vi "readpdf_8.6.vi"(2 "error in (no error)":errorcluster, 3 "Path":path=path "D:/dTemp/Hello World.pdf") -> (0 "error out":errorcluster, 1 "src":string)   [LabVIEW 2012]
uses:
  C:/Users/jlarrieux/Documents/Labview Git Repo/Labview Toolbox/PDFBox.NET-1.7.0/bin/pdfbox-1.7.0.dll
  PDFBox.NET-1.7.0/bin/pdfbox-1.7.0.dll
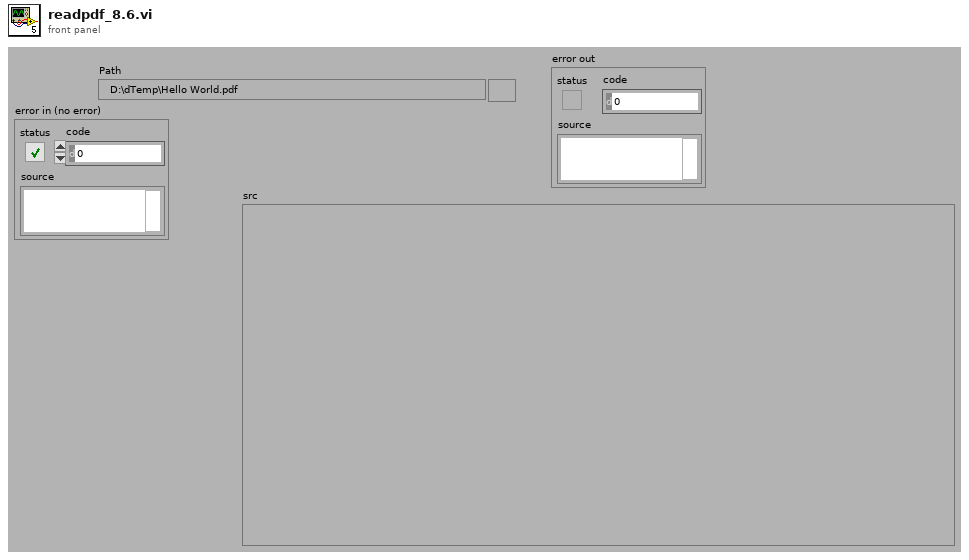
[diagram p1: front panel]
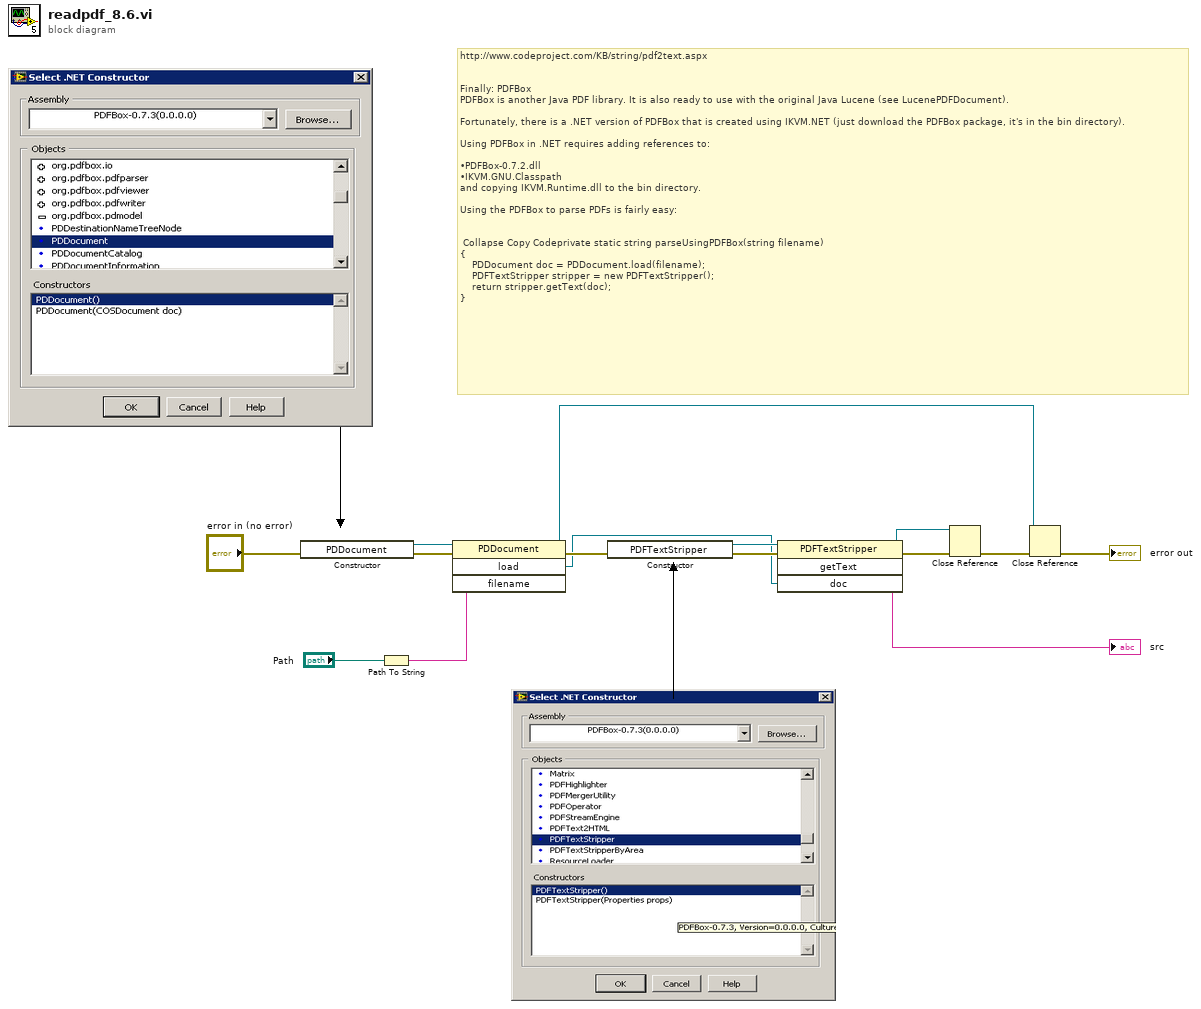
[diagram p0: block diagram]
diagram:
  # "http://www.codeproject.com/KB/string/pdf2text.aspx\n\n\nFinally: PDFBox\nPDFBox is another Java PDF library. It is also ready to use with the original Java Lucene (see LucenePDFDocument).\n\nFortunately, there is a .NET version of PDFBox that is created using IKVM.NET (just download the PDFBox package, it's in the bin directory).\n\nUsing PDFBox in .NET requires adding references to:\n\n•PDFBox-0.7.2.dll \n•IKVM.GNU.Classpath \nand copying IKVM.Runtime.dll to the bin directory.\n\nUsing the PDFBox to parse PDFs is fairly easy:\n\n\n Collapse Copy Codeprivate static string parseUsingPDFBox(string filename)\n{\n    PDDocument doc = PDDocument.load(filename);\n    PDFTextStripper stripper = new PDFTextStripper();\n    return stripper.getText(doc);\n}"
  n1 = constructor class="PDDocument"(error in="error in (no error)") -> (reference out=w15:refnum<k24>, error out=w14:errorcluster)  [unwired: 2 in, 1 out]
  n2 = Path To String(path="Path") -> (string=w12:string)
  n3 = invoke class="PDDocument" method="load"(reference=w15, error in=w14, "filename"=w12) -> (reference out=w3:refnum<k24>, error out=w11:errorcluster, "load"=w2:refnum<k24>)  [unwired: 1 in, 1 out]
  n4 = constructor class="PDFTextStripper"(error in=w11) -> (reference out=w9:refnum<k24>, error out=w10:errorcluster)  [unwired: 2 in, 1 out]
  n5 = invoke class="PDFTextStripper" method="getText"(reference=w9, error in=w10, "doc"=w2) -> (reference out=w6:refnum<k24>, error out=w8:errorcluster, "getText"=→"src":string)  [unwired: 1 in, 1 out]
  n6 = Close Reference(reference=w6, error in (no error)=w8) -> (error out=w7:errorcluster)
  n7 = Close Reference(reference=w3, error in (no error)=w7) -> (error out=→"error out":errorcluster)
